vi "Target State Initialization.vi"(10 "error in (no error)":errorcluster) -> (2 "error out":errorcluster)   [LabVIEW 2018]
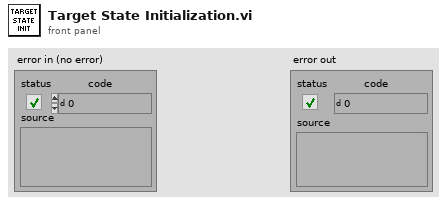
[diagram p1: front panel]
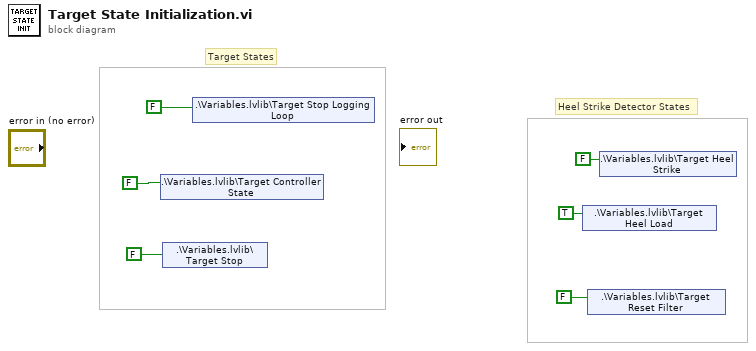
[diagram p0: block diagram]
diagram:
  # "Heel Strike Detector States"
  # "Target States"
  n1 = shared-variable ".\\Variables.lvlib\\Target Controller State"(FALSE ("Target Controller State")) -> ()  [unwired: 1 in, 1 out]
  n2 = shared-variable ".\\Variables.lvlib\\Target Stop"(FALSE ("Target Stop")) -> ()  [unwired: 1 in, 1 out]
  n3 = shared-variable ".\\Variables.lvlib\\Target Stop Logging Loop"(FALSE ("Target Controller State")) -> ()  [unwired: 1 in, 1 out]
  n4 = shared-variable ".\\Variables.lvlib\\Target Heel Load"(TRUE ("Target Heel Load")) -> ()  [unwired: 1 in, 1 out]
  n5 = shared-variable ".\\Variables.lvlib\\Target Reset Filter"(FALSE ("Target Reset Filter")) -> ()  [unwired: 1 in, 1 out]
  n6 = shared-variable ".\\Variables.lvlib\\Target Heel Strike"(FALSE ("Heel Strike?")) -> ()  [unwired: 1 in, 1 out]
